vi "database2查询.vi"(7 "时间2":string, 8 "error in (no error)":errorcluster, 9 "table":string, 10 "时间1":string, 11 "database":string="database1.mdb") -> (0 "error out":errorcluster, 1 "database溢出":bool, 2 "data":string[][](table), 3 "recordset data":variant[][](array[variant]))   [LabVIEW 2016, in "数据传输系统.lvlib"]
uses:
  <vilib>/Utility/sysdir.llb/System Directory Type.ctl
  <vilib>/addons/database/Connection.llb/DB Tools Open Connec (String).vi
  <vilib>/addons/database/Connection.llb/Conn Execute.vi
  <vilib>/addons/database/Recordset.llb/Rec Fetch Recordset Data (R).vi
  <vilib>/addons/database/Recordset.llb/Rec Destroy - Connection.vi
  <vilib>/addons/database/_DB Variant To Data/Database Variant To Data.xnode
  <vilib>/addons/database/NI_Database_API.lvlib
panel:
  out "data 2":string[][](array[string])
  out "仪器代号":string[](array[string])
  out "连接的字符串":string
  out "结果字符串":string
  out "SQL query":string
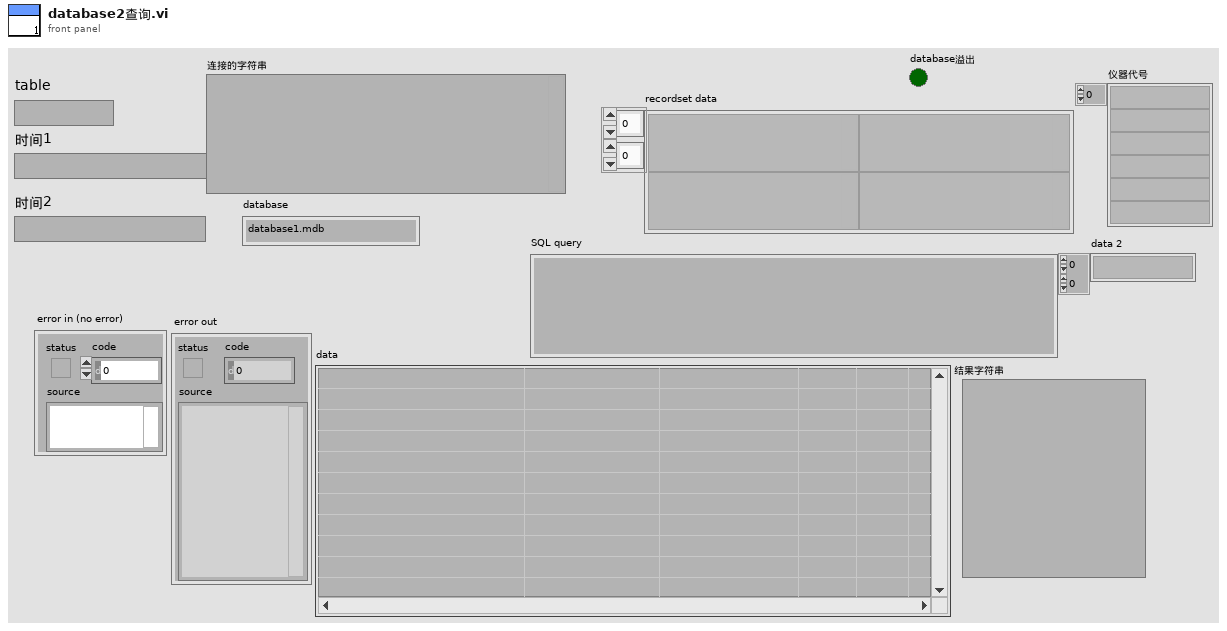
[diagram p1: front panel]
types:
  T1 = typedef "System Directory Type.ctl" = i32
  T2 = typedef "NI_Database_API.lvlib/Conn ObjectReference.ctl" = refnum<k1>
  T3 = typedef "NI_Database_API.lvlib/Rec ObjectReference.ctl" = refnum<k1>
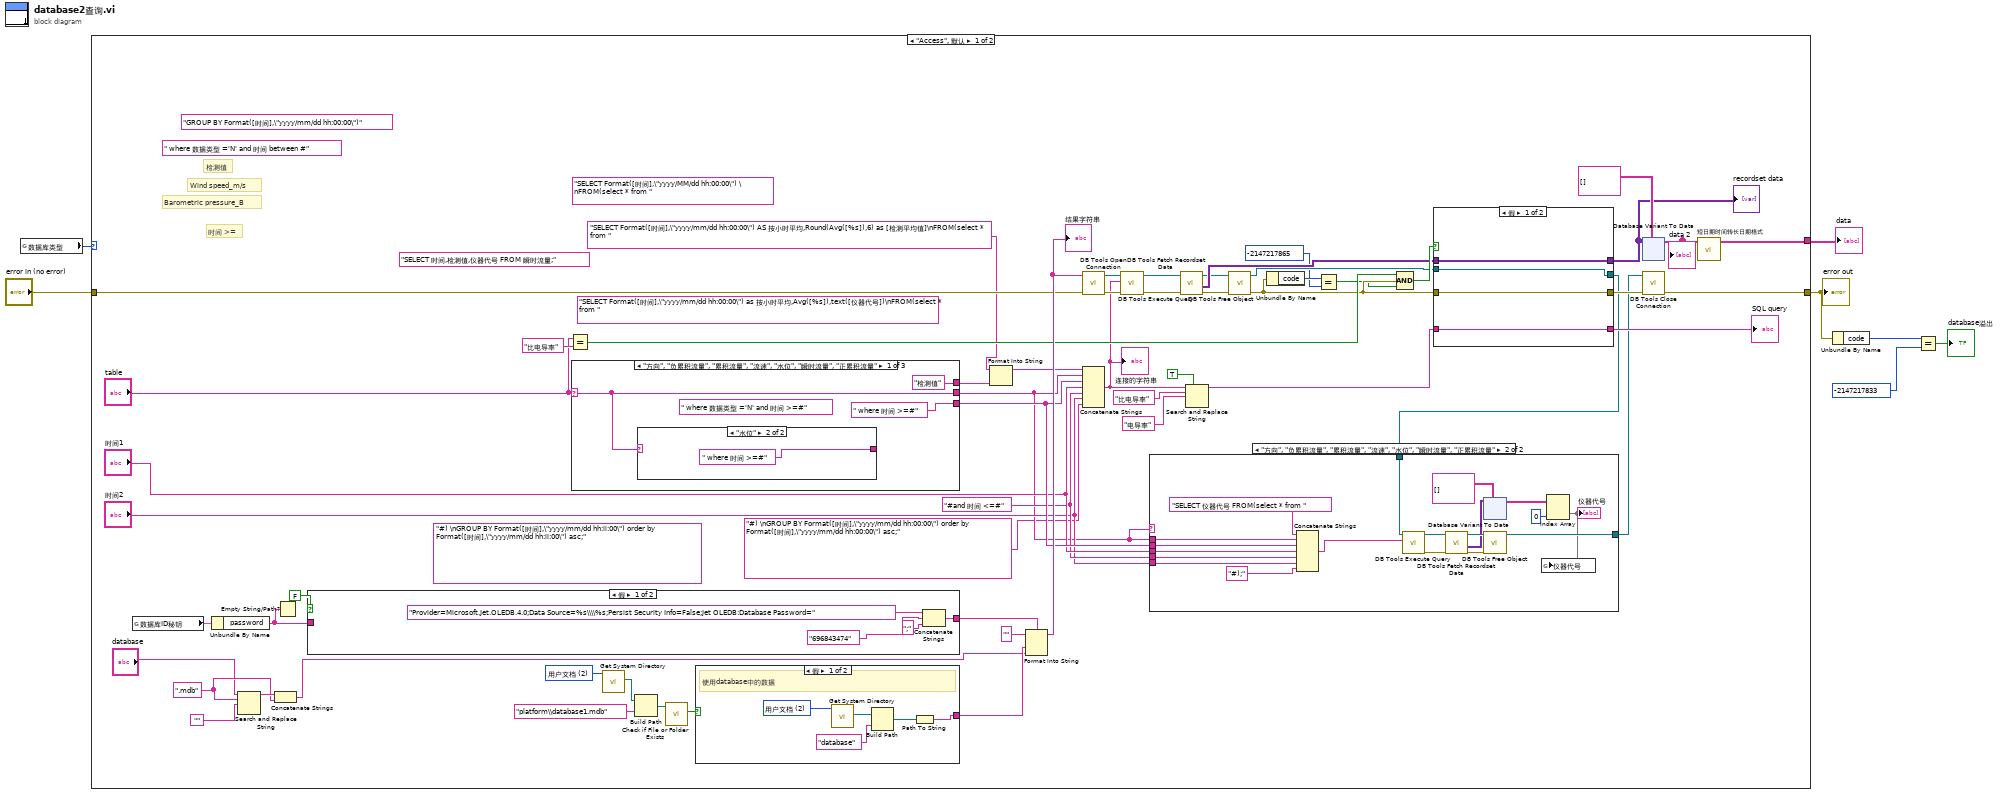
[diagram p0: block diagram]
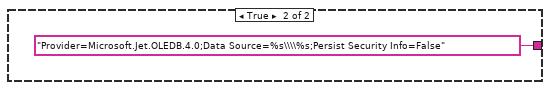
[diagram p3: hidden frame]
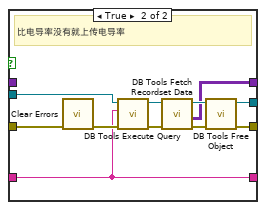
[diagram p4: hidden frame]
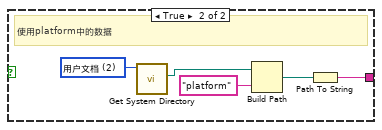
[diagram p5: hidden frame]
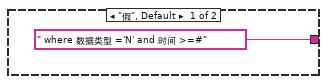
[diagram p6: hidden frame]
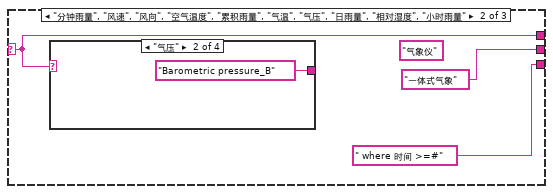
[diagram p7: hidden frame]
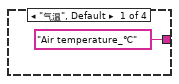
[diagram p8: hidden frame]
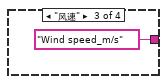
[diagram p9: hidden frame]
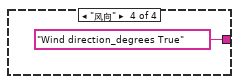
[diagram p10: hidden frame]
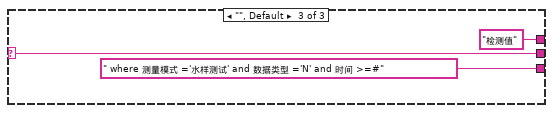
[diagram p11: hidden frame]
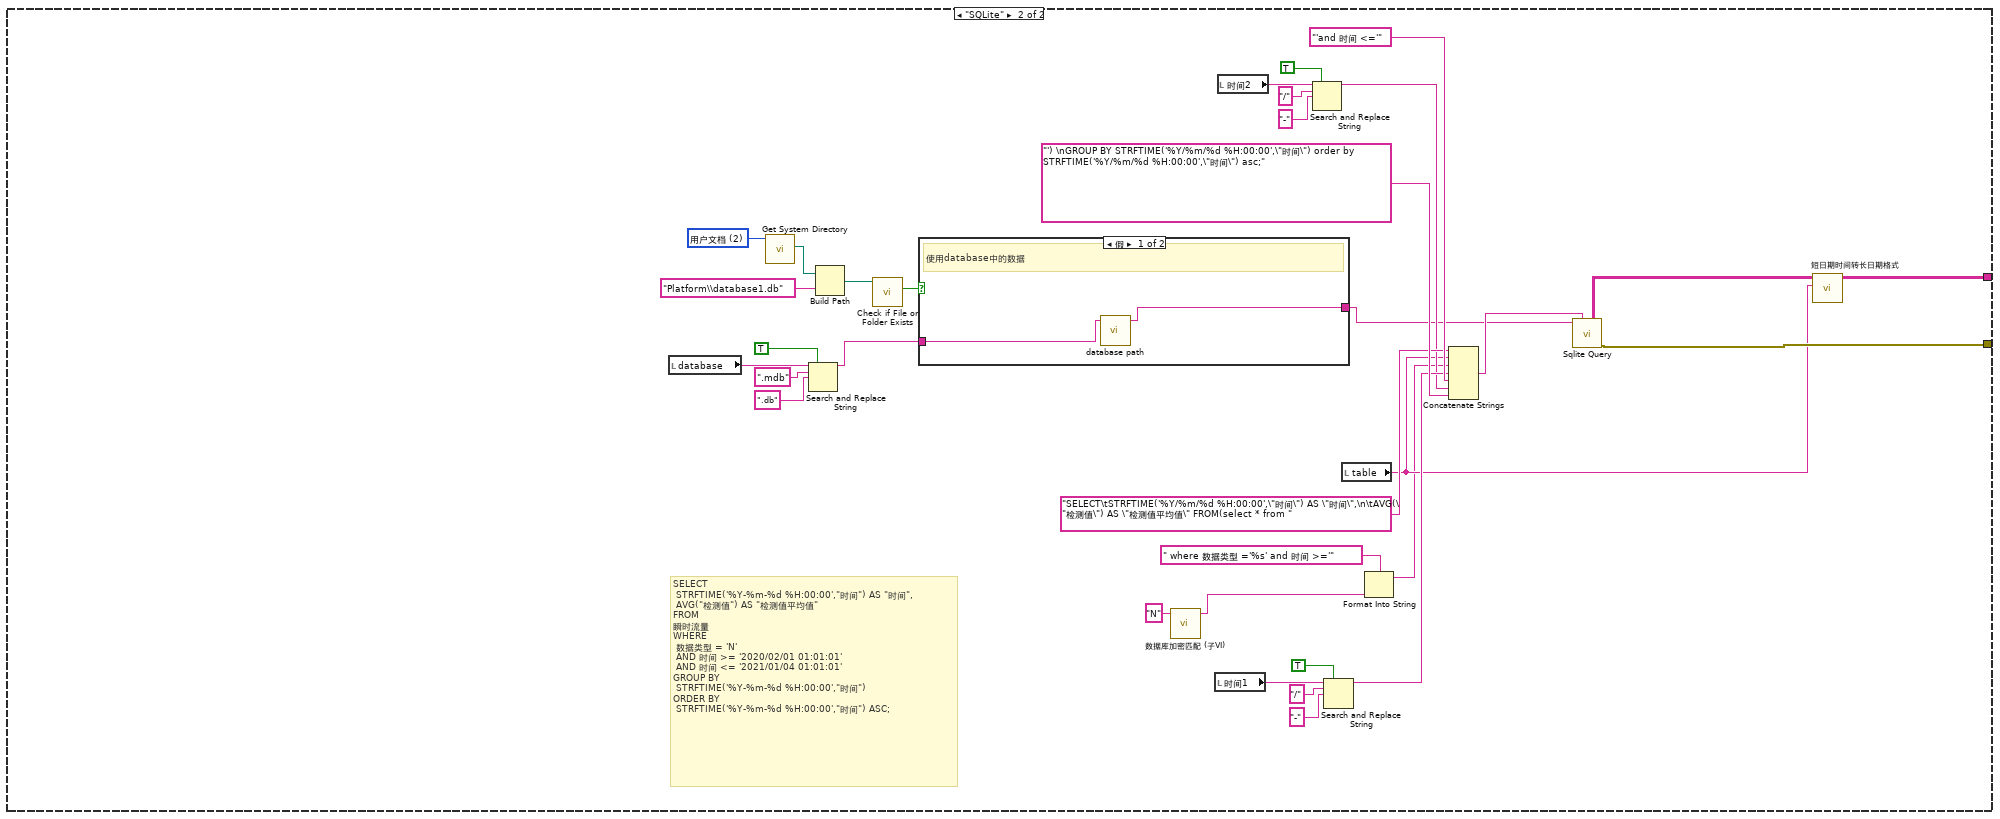
[diagram p12: hidden frame]
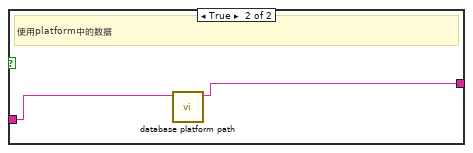
[diagram p13: hidden frame]
diagram:
  n1 = global read "断电保存全局.vi" "数据库类型"() -> (w7:enum16{"Access", "SQLite"})
  n2 = case shown="\"Access\", 默认" w7 {
    tunnel: [w30 w227] -> w4
    tunnel: "error in (no error)" -> [w29 _]
    tunnel: [w24 w243] -> w5
    frame "Access", Default {
      (unwired) "SELECT Format([时间],\"yyyy/MM/dd hh:00:00\") \nFROM(select * from "
      (unwired) "#) \nGROUP BY Format([时间],\"yyyy/mm/dd hh:ii:00\") order by Format([时间],\"yyyy/mm/dd hh:ii:00\") asc;" ("字符串")
      (unwired) "SELECT 时间,检测值,仪器代号 FROM 瞬时流量;" ("连接的字符串")
      w21 = ".mdb" ("搜索字符串")
      (unwired) " where 数据类型 ='N' and 时间 between #"
      w60 = T1 2 items=["用户目录"=0, "用户桌面"=1, "用户文档"=2, "用户应用程序数据"=3, "用户设置"=4, "用户临时目录"=5, "公共文档"=6, "公共应用程序数据"=7, "公共设置"=8, "公共缓存"=13, "系统核心库"=9, "系统安装库"=10, "应用程序文件"=11, "启动盘根目录"=12] ("system directory type")
      (unwired) "GROUP BY Format([时间],\"yyyy/mm/dd hh:00:00\")"
      w14 = "#and 时间 <=#"
      (unwired) "SELECT Format([时间],\"yyyy/mm/dd hh:00:00\") as 按小时平均,Avg([%s]),text([仪器代号])\nFROM(select * from "
      # "时间 >="
      # "Wind speed_m/s"
      # "检测值"
      # "Barometric pressure_B"
      n3 = global read "外部交互全局.vi" "数据库ID秘钥"() -> (w31:cluster{"userID":string, "password":string})
      n4 = Unbundle By Name(w31) -> ("password"=w33:string)
      n5 = Search and Replace String(input string="database", search string=w21, replace string="") -> (result string=w22:string)  [unwired: 5 in, 3 out]
      n6 = Concatenate Strings(w22, w21) -> (w19:string)
      n7 = Empty String/Path?(string/path=w33) -> ()  [unwired: 1 out]
      n8 = case shown="假" FALSE {
        tunnel: [w174 "Provider=Microsoft.Jet.OLEDB.4.0;Data Source=%s\\\\%s;Persist Security Info=False" ("格式字符串")] -> w32
        tunnel: w33 -> [_ _]
        frame False {
          n9 = Concatenate Strings("Provider=Microsoft.Jet.OLEDB.4.0;Data Source=%s\\\\%s;Persist Security Info=False;Jet OLEDB:Database Password=" ("格式字符串"), "696843474" ("格式字符串"), ";" ("字符串")) -> (w174:string)
        }
        frame True {
        }
      }
      n10 = Equal?(x="table", y="比电导率") -> (x = y?=w49:bool)
      n11 = case shown="\"方向\", \"负累积流量\", \"累积流量\", \"流速\", \"水位\", \"瞬时流量\", \"正累积流量\"" "table" {
        selector: "table" -> [w204 w208 w216]
        tunnel: [" where 时间 >=#" " where 时间 >=#" " where 测量模式 ='水样测试' and 数据类型 ='N' and 时间 >=#"] -> w16
        tunnel: ["检测值" w208 "检测值"] -> w36
        tunnel: [w204 "一体式气象" w216] -> w11
        frame "方向", "负累积流量", "累积流量", "流速", "水位", "瞬时流量", "正累积流量" {
          (unwired) " where 数据类型 ='N' and 时间 >=#"
          n12 = case shown="\"水位\"" w204 {
            tunnel: [" where 数据类型 ='N' and 时间 >=#" " where 时间 >=#"] -> _
            frame "假", Default {
            }
            frame "水位" {
            }
          }
        }
        frame "分钟雨量", "风速", "风向", "空气温度", "累积雨量", "气温", "气压", "日雨量", "相对湿度", "小时雨量" {
          (unwired) "气象仪"
          n13 = case shown="\"气压\"" w208 {
            tunnel: ["Air temperature_℃" "Barometric pressure_B" "Wind speed_m/s" "Wind direction_degrees True"] -> _
            frame "气温", Default {
            }
            frame "气压" {
            }
            frame "风速" {
            }
            frame "风向" {
            }
          }
        }
        frame "", Default {
        }
      }
      n14 = call <vilib>:"Get System Directory.vi"("system directory type"=w60) -> ("system directory"=w61:path)  [unwired: 10 in]
      n15 = Build Path(base path=w61, name or relative path="platform\\database1.mdb" ("condition")) -> (appended path=w59:path)
      n16 = call <vilib>:"Check if File or Folder Exists.vi"("path"=w59) -> ("file or folder exists?"=w57:bool)  [unwired: 8 in, 2 out]
      n17 = case shown="假" w57 {
        tunnel: [w193 w198] -> w56
        frame False {
          w196 = T1 2 items=["用户目录"=0, "用户桌面"=1, "用户文档"=2, "用户应用程序数据"=3, "用户设置"=4, "用户临时目录"=5, "公共文档"=6, "公共应用程序数据"=7, "公共设置"=8, "公共缓存"=13, "系统核心库"=9, "系统安装库"=10, "应用程序文件"=11, "启动盘根目录"=12] ("system directory type")
          # "使用database中的数据"
          n18 = call <vilib>:"Get System Directory.vi"("system directory type"=w196) -> ("system directory"=w195:path)  [unwired: 10 in]
          n19 = Build Path(base path=w195, name or relative path="database" ("condition")) -> (appended path=w197:path)
          n20 = Path To String(path=w197) -> (string=w193:string)
        }
        frame True {
          w202 = T1 2 items=["用户目录"=0, "用户桌面"=1, "用户文档"=2, "用户应用程序数据"=3, "用户设置"=4, "用户临时目录"=5, "公共文档"=6, "公共应用程序数据"=7, "公共设置"=8, "公共缓存"=13, "系统核心库"=9, "系统安装库"=10, "应用程序文件"=11, "启动盘根目录"=12] ("system directory type")
          # "使用platform中的数据"
          n21 = call <vilib>:"Get System Directory.vi"("system directory type"=w202) -> ("system directory"=w201:path)  [unwired: 10 in]
          n22 = Build Path(base path=w201, name or relative path="platform" ("condition")) -> (appended path=w199:path)
          n23 = Path To String(path=w199) -> (string=w198:string)
        }
      }
      n24 = Format Into String(initial string="SELECT Format([时间],\"yyyy/mm/dd hh:00:00\") AS 按小时平均,Round(Avg([%s]),6) as [检测平均值]\nFROM(select * from ", w36) -> (resulting string=w34:string)  [unwired: 2 in, 1 out]
      n25 = Format Into String(format string=w32, initial string="" ("初始字符串"), w56, w19) -> (resulting string=w55:string)  [unwired: 1 in, 1 out]
      "结果字符串" <- w55
      n26 = call-poly <vilib>:"DB Tools Open Connection.vi"("error in (no error)"=w29, "connection information"=w55) -> ("error out"=w63:errorcluster, "connection reference"=w51:T2)  [unwired: 6 in]
      n27 = Concatenate Strings(w34, w11, w16, "时间1", w14, "时间2", "#) \nGROUP BY Format([时间],\"yyyy/mm/dd hh:00:00\") order by Format([时间],\"yyyy/mm/dd hh:00:00\") asc;" ("字符串")) -> (w18:string)
      "连接的字符串" <- w18
      n28 = call-poly <vilib>:"DB Tools Execute Query.vi"("error in (no error)"=w63, "SQL query"=w18, "connection reference"=w51) -> ("error out"=w47:errorcluster, "recordset reference"=w52:T3)  [unwired: 5 in]
      n29 = call-poly <vilib>:"DB Tools Fetch Recordset Data.vi"("error in (no error)"=w47, "recordset reference"=w52) -> ("error out"=w64:errorcluster, "recordset data"=w53:variant[][], "recordset reference out"=w48:T3)  [unwired: 3 in]
      n30 = Search and Replace String(replace all?=TRUE ("替换全部？(F)"), input string=w18, search string="比电导率" ("搜索字符串"), replace string="电导率" ("替换字符串(\"\")")) -> (result string=w39:string)  [unwired: 4 in, 3 out]
      n31 = call-poly <vilib>:"DB Tools Free Object.vi"("error in (no error)"=w64, "recordset reference"=w48) -> ("error out"=w43:errorcluster, "connection reference"=w46:T2)  [unwired: 8 in]
      n32 = Unbundle By Name(w43) -> ("code"=w45:i32)
      n33 = Equal?(x=w45, y=-2147217865 ("code")) -> (x = y?=w42:bool)
      n34 = Compound Arithmetic op=AND ("复合运算")(w49, w43, w42) -> (w54:bool)
      n35 = case shown="假" w54 {
        tunnel: w39 -> [w178 w182]
        tunnel: w46 -> [w179 w187]
        tunnel: [w179 w183] -> w17
        tunnel: [w181 w185] -> w25
        tunnel: w53 -> [w181 _]
        tunnel: w43 -> [w180 w192]
        tunnel: [w180 w184] -> w26
        tunnel: [w178 w182] -> w37
        frame False {
        }
        frame True {
          # "比电导率没有就上传电导率"
          n36 = call <vilib>:"Clear Errors.vi"("error in (no error)"=w192) -> ("error out"=w186:errorcluster)  [unwired: 5 in, 1 out]
          n37 = call-poly <vilib>:"DB Tools Execute Query.vi"("error in (no error)"=w186, "SQL query"=w182, "connection reference"=w187) -> ("error out"=w188:errorcluster, "recordset reference"=w190:T3)  [unwired: 5 in]
          n38 = call-poly <vilib>:"DB Tools Fetch Recordset Data.vi"("error in (no error)"=w188, "recordset reference"=w190) -> ("error out"=w191:errorcluster, "recordset data"=w185:variant[][], "recordset reference out"=w189:T3)  [unwired: 3 in]
          n39 = call-poly <vilib>:"DB Tools Free Object.vi"("error in (no error)"=w191, "recordset reference"=w189) -> ("error out"=w184:errorcluster, "connection reference"=w183:T2)  [unwired: 8 in]
        }
      }
      "SQL query" <- w37
      "recordset data" <- w25
      n40 = case shown="\"方向\", \"负累积流量\", \"累积流量\", \"流速\", \"水位\", \"瞬时流量\", \"正累积流量\"" w11 {
        tunnel: w17 -> [w65 w80]
        tunnel: w11 -> [_ w79]
        tunnel: w16 -> [_ w78]
        tunnel: "时间1" -> [_ w77]
        tunnel: w14 -> [_ w76]
        tunnel: "时间2" -> [_ w75]
        tunnel: [w65 w71] -> w12
        frame "假", Default {
        }
        frame "方向", "负累积流量", "累积流量", "流速", "水位", "瞬时流量", "正累积流量" {
          n41 = Concatenate Strings("SELECT 仪器代号 FROM(select * from " ("连接的字符串"), w79, w78, w77, w76, w75, "#);" ("连接的字符串")) -> (w72:string)
          n42 = call-poly <vilib>:"DB Tools Execute Query.vi"("SQL query"=w72, "connection reference"=w80) -> ("error out"=w84:errorcluster, "recordset reference"=w82:T3)  [unwired: 6 in]
          n43 = call-poly <vilib>:"DB Tools Fetch Recordset Data.vi"("error in (no error)"=w84, "recordset reference"=w82) -> ("error out"=w81:errorcluster, "recordset data"=w70:variant[][], "recordset reference out"=w83:T3)  [unwired: 3 in]
          n44 = xnode "Database Variant To Data"("database variant"=w70, "type"=string[][] []) -> ("data"=w68:string[][])  [unwired: 1 in, 1 out]
          n45 = call-poly <vilib>:"DB Tools Free Object.vi"("error in (no error)"=w81, "recordset reference"=w83) -> ("connection reference"=w71:T2)  [unwired: 8 in, 1 out]
          n46 = Index Array(array=w68, index (col)=0 ("禁用的索引 (列)")) -> (element=w66:string[])  [unwired: 1 in]
          "仪器代号" <- w66
          n47 = global write "全局 所有参数.vi" "仪器代号"(w66) -> ()
        }
      }
      n48 = xnode "Database Variant To Data"("database variant"=w25, "type"=string[][] []) -> ("data"=w27:string[][])  [unwired: 1 in, 1 out]
      "data 2" <- w27
      n49 = call <vilib>:"DB Tools Close Connection.vi"("error in (no error)"=w26, "connection reference"=w12) -> ("error out"=w30:errorcluster)  [unwired: 5 in]
      n50 = call "短日期时间转长日期格式.vi"("data"=w27) -> ("输出数组"=w24:string[][])  [unwired: 10 in]
    }
    frame "SQLite" {
      w247 = T1 2 items=["用户目录"=0, "用户桌面"=1, "用户文档"=2, "用户应用程序数据"=3, "用户设置"=4, "用户临时目录"=5, "公共文档"=6, "公共应用程序数据"=7, "公共设置"=8, "公共缓存"=13, "系统核心库"=9, "系统安装库"=10, "应用程序文件"=11, "启动盘根目录"=12] ("system directory type")
      # "SELECT\n\tSTRFTIME('%Y-%m-%d %H:00:00',\"时间\") AS \"时间\",\n\tAVG(\"检测值\") AS \"检测值平均值\"\nFROM\n瞬时流量 \nWHERE\n\t数据类型 = 'N' \n\tAND 时间 >= '2020/02/01 01:01:01' \n\tAND 时间 <= '2021/01/04 01:01:01' \nGROUP BY\n\tSTRFTIME('%Y-%m-%d %H:00:00',\"时间\")\nORDER BY\n\tSTRFTIME('%Y-%m-%d %H:00:00',\"时间\") ASC;"
      n51 = local read "database"() -> (w228:string)
      n52 = call <vilib>:"Get System Directory.vi"("system directory type"=w247) -> ("system directory"=w246:path)  [unwired: 10 in]
      n53 = Search and Replace String(replace all?=TRUE ("替换全部？(F)"), input string=w228, search string=".mdb" ("搜索字符串"), replace string=".db" ("替换字符串(\"\")")) -> (result string=w219:string)  [unwired: 4 in, 3 out]
      n54 = Build Path(base path=w246, name or relative path="Platform\\database1.db" ("condition")) -> (appended path=w248:path)
      n55 = call <vilib>:"Check if File or Folder Exists.vi"("path"=w248) -> ("file or folder exists?"=w250:bool)  [unwired: 8 in, 2 out]
      n56 = case shown="假" w250 {
        tunnel: [w251 w253] -> w218
        tunnel: w219 -> [w252 w254]
        frame False {
          # "使用database中的数据"
          n57 = call "database path.vi"("database"=w252) -> ("Path out"=w251:string)  [unwired: 9 in, 1 out]
        }
        frame True {
          # "使用platform中的数据"
          n58 = call "database platform path.vi"("database"=w254) -> ("Path out"=w253:string)  [unwired: 10 in]
        }
      }
      n59 = call "数据库加密匹配 (子VI).vi"("输入参数"="N") -> ("Encoded String"=w221:string)  [unwired: 10 in]
      n60 = local read "时间1"() -> (w235:string)
      n61 = local read "时间2"() -> (w233:string)
      n62 = Search and Replace String(replace all?=TRUE ("替换全部？(F)"), input string=w233, search string="/" ("搜索字符串"), replace string="-" ("替换字符串(\"\")")) -> (result string=w232:string)  [unwired: 4 in, 3 out]
      n63 = Search and Replace String(replace all?=TRUE ("替换全部？(F)"), input string=w235, search string="/" ("搜索字符串"), replace string="-" ("替换字符串(\"\")")) -> (result string=w234:string)  [unwired: 4 in, 3 out]
      n64 = local read "table"() -> (w225:string)
      n65 = Format Into String(format string=" where 数据类型 ='%s' and 时间 >='", w221) -> (resulting string=w223:string)  [unwired: 2 in, 1 out]
      n66 = Concatenate Strings("SELECT\tSTRFTIME('%Y/%m/%d %H:00:00',\"时间\") AS \"时间\",\n\tAVG(\"检测值\") AS \"检测值平均值\" FROM(select * from ", w225, w223, w234, "'and 时间 <='", w232, "') \nGROUP BY STRFTIME('%Y/%m/%d %H:00:00',\"时间\") order by STRFTIME('%Y/%m/%d %H:00:00',\"时间\") asc;" ("字符串")) -> (w220:string)
      n67 = call "Sqlite Query.vi"("DB Path"=w218, "SQL Query"=w220) -> ("Results"=w226:string[][], "error out"=w227:errorcluster)  [unwired: 11 in, 1 out]
      n68 = call "短日期时间转长日期格式.vi"("table输入"=w225, "data"=w226) -> ("输出数组"=w243:string[][])  [unwired: 9 in]
    }
  }
  "error out" <- w4
  "data" <- w5
  n69 = Unbundle By Name(w4) -> ("code"=w3:i32)
  n70 = Equal?(x=w3, y=-2147217833 ("code")) -> (x = y?=→"database溢出":bool)
